vi "Close JKI SM for Tests.vi"(8 "error in (no error)":errorcluster, 11 "JKI SM in":refnum<class "JKI SM.lvclass">) -> (0 "error out":errorcluster)   [LabVIEW 2013, in "JKI State Machine API - Tests.lvlib"]
uses:
  JKI State Machine API - Tests.lvlib
  source/JKI SM/JKI SM.lvclass
  source/JKI SM/JKI SM.lvclass/JKI SM.ctl
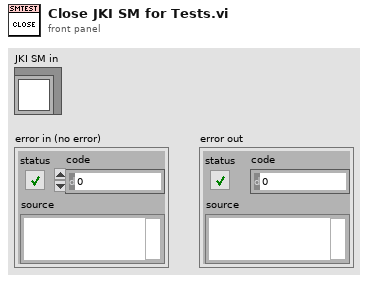
[diagram p1: front panel]
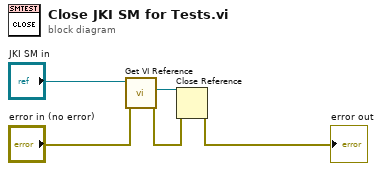
[diagram p0: block diagram]
diagram:
  n1 = call "Get VI Reference.vi"("error in (no error)"="error in (no error)", "JKI SM in"="JKI SM in") -> ("error out"=w1:errorcluster, "VI"=w4:refnum<vi>)  [unwired: 7 in, 1 out]
  n2 = Close Reference(reference=w4, error in (no error)=w1) -> (error out=→"error out":errorcluster)
